vi "Read Field - I16.vi"(7 "field name":string, 8 "error in (no error)":errorcluster, 10 "default":i16, 11 "PV Data in":refnum<class "PV Data.lvclass">) -> (0 "error out":errorcluster, 2 "value":i16, 3 "PV Data out":refnum<class "PV Data.lvclass">)   [LabVIEW 2020, in "PV Access.lvlib" / "PV Data.lvlib" / "PV Data.lvclass"]
uses:
  PV Data.lvclass
  PV Access.lvlib
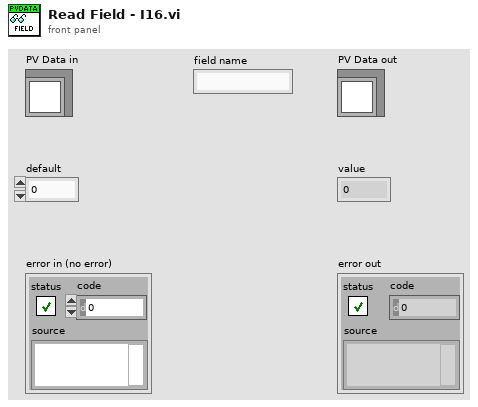
[diagram p1: front panel]
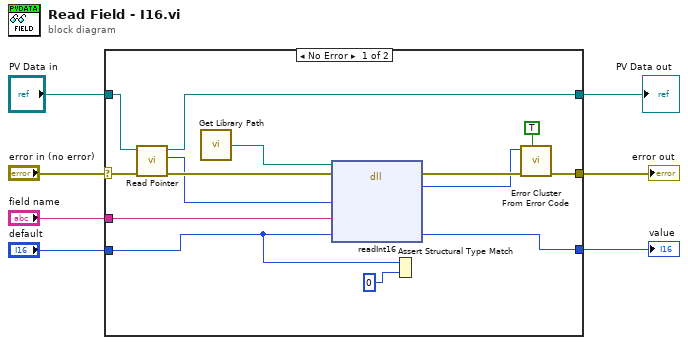
[diagram p0: block diagram]
diagram:
  n1 = case shown="No Error" "error in (no error)" {
    selector: "error in (no error)" -> [w14 w24]
    tunnel: [w15 w24] -> w7
    tunnel: "PV Data in" -> [w12 w23]
    tunnel: [w10 w23] -> w2
    tunnel: "default" -> [w21 w22]
    tunnel: [w20 w22] -> w4
    tunnel: "field name" -> [w9 _]
    frame No Error {
      n2 = call-dynamic "Read Pointer.vi"("error in (no error)"=w14, "Pointer Base in"=w12) -> ("error out"=w13:errorcluster, "Pointer"=w11:i64, "Pointer Base out"=w10:refnum<class "PV Data.lvclass">)  [unwired: 7 in]
      n3 = call "Get Library Path.vi"() -> ("Path"=w19:path)  [unwired: 1 in]
      n4 = dll-call lib="?" fn="readInt16"(path in=w19, error in=w13, "value"=w11, "field_name"=w9, "result"=w21) -> (error out=w17:errorcluster, "err_code"=w16:i32, "result"=w20:i16)  [unwired: 3 in, 1 out]
      n5 = Assert Structural Type Match(0:i16 0, 1:w21) -> ()
      n6 = call <vilib>:"Error Cluster From Error Code.vi"("show call chain? (False)"=TRUE, "error in (no error)"=w17, "error code (0)"=w16) -> ("error out"=w15:errorcluster)  [unwired: 6 in]
    }
    frame Error {
    }
  }
  "error out" <- w7
  "value" <- w4
  "PV Data out" <- w2
